vi "Sensor Simulation Initialization VI.vi"(8 "error in (no error)":errorcluster, 10 "Custom XML":string, 11 "Device Item Ref in":T1 format="%.0x") -> (0 "error out":errorcluster, 3 "Device Item Ref out":T1 format="%.0x")   [LabVIEW 2011, in "Sensor Simulation Custom Device.lvlib"]
uses:
  Sensor Simulation Custom Device.lvlib
  <vilib>/NI Veristand/Custom Device API/Custom Device Item Ref.ctl
  <vilib>/NI Veristand/Custom Device API/Dependent File Optional Info.ctl
  Real-Time/TypeDefs/SensorType.ctl
  <vilib>/NI Veristand/Custom Device API/Custom Device Channel.ctl
  <vilib>/NI Veristand/Custom Device API/Custom Device Channel Type.ctl
  Global.vi
  <vilib>/NI Veristand/Custom Device API/Set Item Property (Path).vi
  <vilib>/NI Veristand/Custom Device API/Set Item Property (String).vi
  <vilib>/NI Veristand/Custom Device API/Set Item Property (Boolean).vi
  <vilib>/NI Veristand/Custom Device API/Set Item Property (Dependent Node Pointer).vi
  <vilib>/NI Veristand/Custom Device API/Set Item Property (Dependent File).vi
  <vilib>/NI Veristand/Custom Device API/Set Item Property (Variant).vi
  <vilib>/NI Veristand/Custom Device API/Custom Device API.lvlib
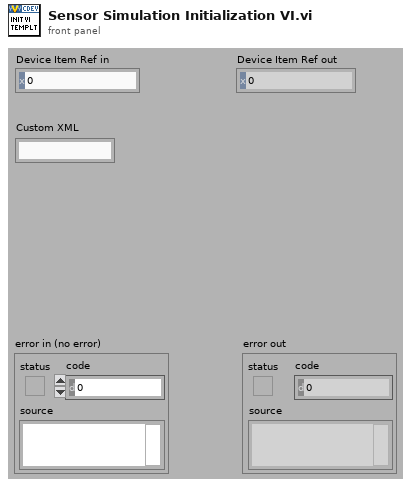
[diagram p1: front panel]
types:
  T1 = typedef "Custom Device API.lvlib/Custom Device Item Ref.ctl" = u64
  T2 = typedef "Sensor Simulation Custom Device.lvlib/SensorType.ctl" = enum16{"Resolver", "4 Wire xVDT", "5 Wire xVDT", "Invalid"}
  T3 = typedef "Custom Device API.lvlib/Custom Device Channel.ctl" = cluster{"Type":T4, "Units":string, "Default Value":dbl, "Faultable":bool, "Scalable":bool}
  T4 = typedef "Custom Device API.lvlib/Custom Device Channel Type.ctl" = enum16{"Input", "Output"}
  T5 = typedef "Custom Device API.lvlib/Dependent File Optional Info.ctl" = cluster{"Version":string, "RTDestination":path, "ForceDownload":bool, "SupportedTarget":string, "MD5":string}
  T6 = typedef "Sensor Simulation Custom Device.lvlib/SensorSimComps.ctl" = cluster{"xVDTs":T7[], "Resolvers":T8[]}
  T7 = typedef "Sensor Simulation Custom Device.lvlib/xVDT.ctl" = cluster{"ScaleFactor 1":string, "ScaleFactor 2":string, "#":string}
  T8 = typedef "Sensor Simulation Custom Device.lvlib/Resolver.ctl" = cluster{"ScaleFactor 1":string, "ScaleFactor 2":string, "#":string}
  T9 = cluster{"RIO Device Address":string, "Bitfile Signature":string, "Engine Sim Components":T6}
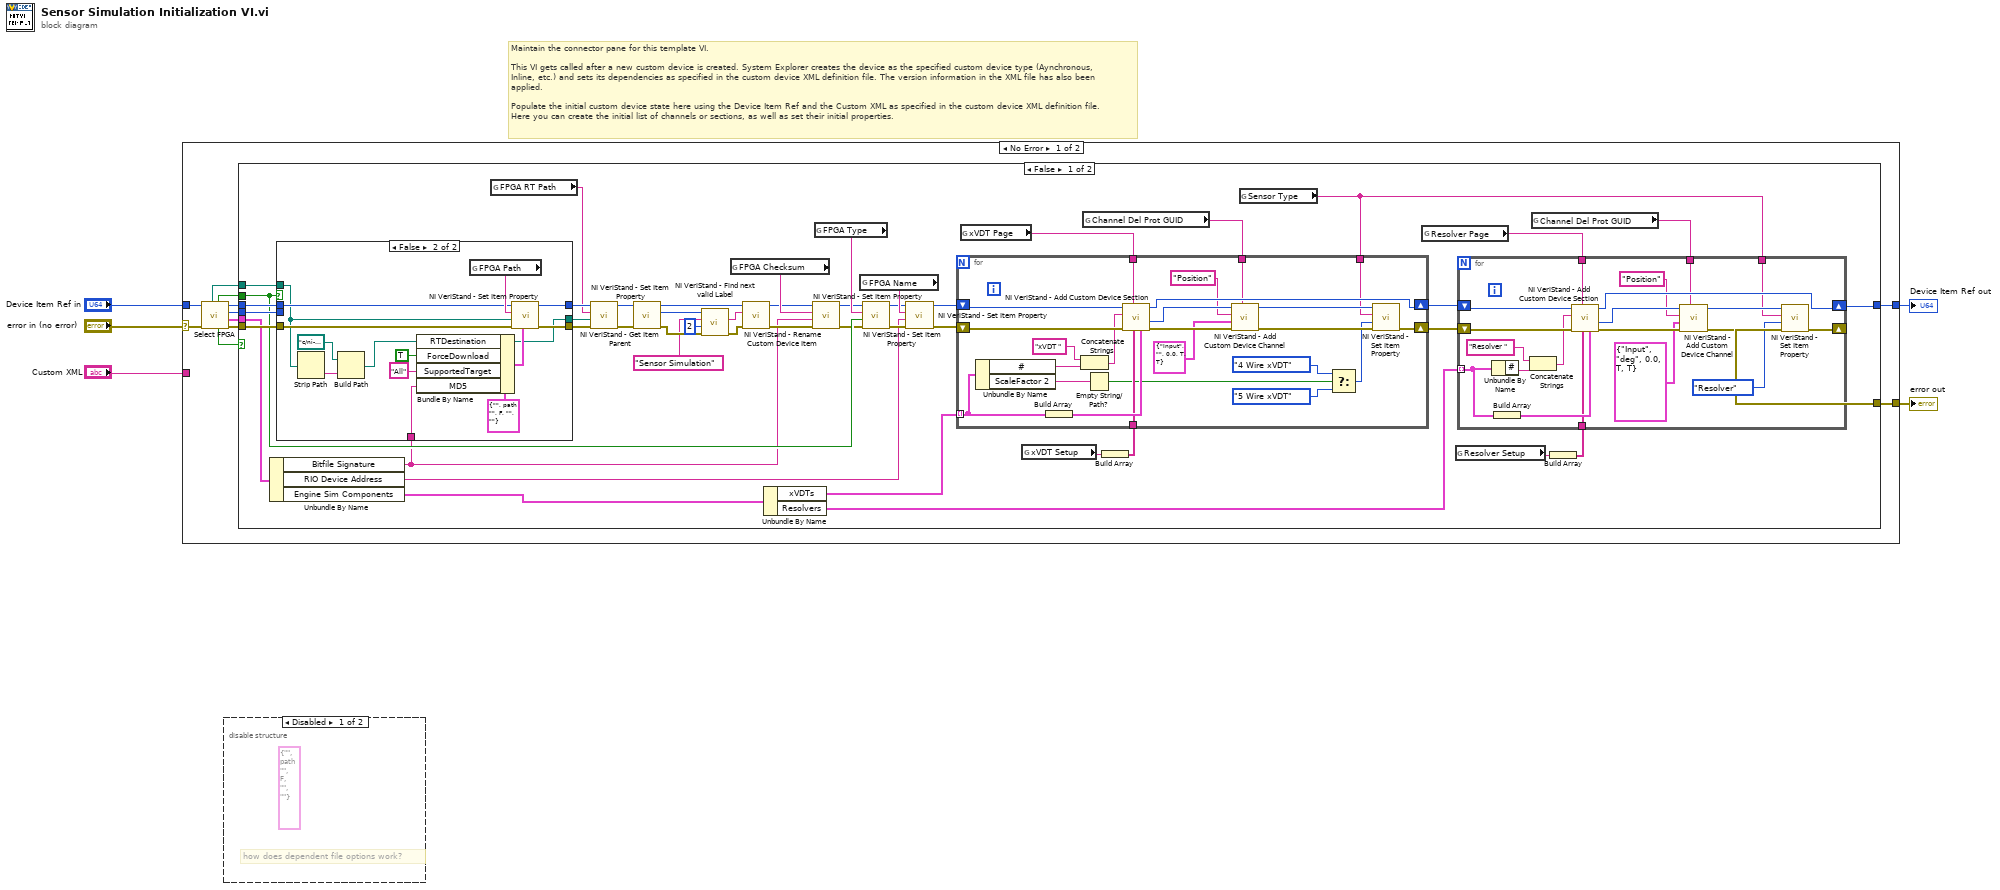
[diagram p0: block diagram]
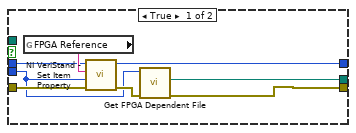
[diagram p3: hidden frame]
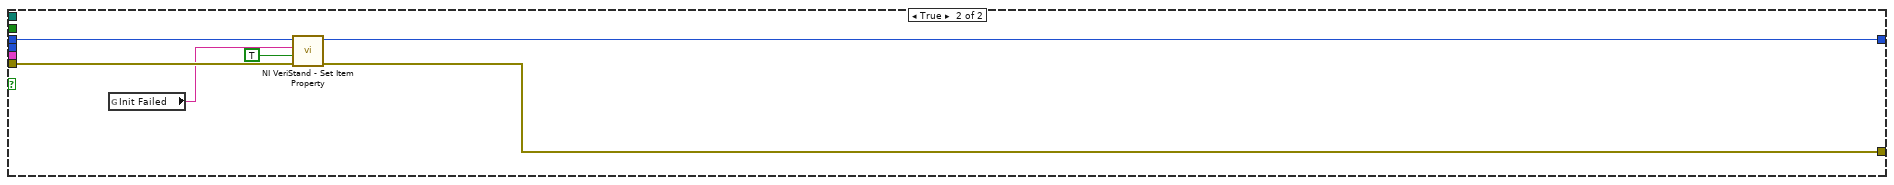
[diagram p4: hidden frame]
diagram:
  # "Maintain the connector pane for this template VI.\n\nThis VI gets called after a new custom device is created. System Explorer creates the device as the specified custom device type (Aynchronous, Inline, etc.) and sets its dependencies as specified in the custom device XML definition file. The version information in the XML file has also been applied.\n\nPopulate the initial custom device state here using the Device Item Ref and the Custom XML as specified in the custom device XML definition file. Here you can create the initial list of channels or sections, as well as set their initial properties."
  n1 = case shown="No Error" "error in (no error)" {
    selector: "error in (no error)" -> [w15 w136]
    tunnel: [w8 w136] -> w5
    tunnel: [w7 w135] -> w3
    tunnel: "Device Item Ref in" -> [w16 w135]
    tunnel: "Custom XML" -> [_ _]
    frame No Error {
      n2 = call "Select FPGA.vi"("error in"=w15, "Item Ref in"=w16) -> ("error out"=w13:errorcluster, "FPGA Info"=w11:T9, "FPGA Reference"=w14:T1, "Item Ref out"=w12:T1, "Cancelled?"=w6:bool, "VS FPGA?"=w10:bool, "Bitfile Path out"=w9:path)  [unwired: 3 in]
      n3 = case shown="False" w6 {
        tunnel: w14 -> [w62 _]
        tunnel: w13 -> [w61 w133]
        tunnel: w12 -> [w60 w134]
        tunnel: w11 -> [w59 _]
        tunnel: w10 -> [w58 _]
        tunnel: w9 -> [w57 _]
        tunnel: [w22 w132] -> w8
        tunnel: [w23 w131] -> w7
        frame False {
          n4 = Unbundle By Name(w59) -> ("Bitfile Signature"=w38:string, "RIO Device Address"=w48:string, "Engine Sim Components"=w56:T6)
          n5 = case shown="False" w58 {
            tunnel: w62 -> [w110 _]
            tunnel: w61 -> [w112 w126]
            tunnel: w60 -> [w113 w127]
            tunnel: w57 -> [_ w123]
            tunnel: [w109 w125] -> w20
            tunnel: [w108 w124] -> w19
            tunnel: w38 -> [_ w116]
            tunnel: [w107 w115] -> w18
            frame True {
              n6 = global read "Global.vi" "FPGA Reference"() -> (w114:string)
              n7 = call-poly <vilib>:"NI VeriStand - Set Item Property.vi"("error in (no error)"=w112, "Dependent Node Ref"=w110, "Property Name"=w114, "Item Ref in"=w113) -> ("error out"=w111:errorcluster, "Item Ref out"=w108:T1)  [unwired: 5 in, 1 out]
              n8 = call "Get FPGA Dependent File.vi"("error in (no error)"=w111, "ID in"=w110) -> ("error out"=w109:errorcluster, "RT Path"=w107:path)  [unwired: 7 in, 1 out]
            }
            frame False {
              n9 = Strip Path(path=w123) -> (name=w122:string)  [unwired: 1 out]
              n10 = Build Path(base path=path "c:/ni-rt/NIVeriStand/Custom Devices/Sensor Simulation" ("RTDestination"), name or relative path=w122) -> (appended path=w115:path)
              n11 = Bundle By Name(cluster=T5 {"Version"="", "RTDestination"=path "", "ForceDownload"=FALSE, "SupportedTarget"="", "MD5"=""} ("OptionalInfo"), "RTDestination"=w115, "ForceDownload"=TRUE, "SupportedTarget"="All", "MD5"=w116) -> (w118:T5)
              n12 = global read "Global.vi" "FPGA Path"() -> (w128:string)
              n13 = call-poly <vilib>:"NI VeriStand - Set Item Property.vi"("OptionalInfo"=w118, "error in (no error)"=w126, "Path"=w123, "Property Name"=w128, "Item Ref in"=w127) -> ("error out"=w125:errorcluster, "Item Ref out"=w124:T1)  [unwired: 4 in, 1 out]
            }
          }
          n14 = global read "Global.vi" "FPGA RT Path"() -> (w17:string)
          n15 = call-poly <vilib>:"NI VeriStand - Set Item Property.vi"("error in (no error)"=w20, "Value"=w18, "Property Name"=w17, "Item Ref in"=w19) -> ()  [unwired: 5 in, 3 out]
          n16 = call <vilib>:"NI VeriStand - Get Item Parent.vi"("error in (no error)"=w20, "Item Ref in"=w19) -> ("error out"=w42:errorcluster, "Parent Ref"=w44:T1, "Item Ref out"=w45:T1)  [unwired: 6 in, 1 out]
          n17 = call <vilib>:"NI VeriStand - Find next valid Label.vi"("error in (no error)"=w42, "Start Value (1)"=2, "Label"="Sensor Simulation", "Item Ref in"=w44) -> ("error out"=w41:errorcluster, "Label out"=w43:string)  [unwired: 3 in, 3 out]
          n18 = global read "Global.vi" "FPGA Checksum"() -> (w51:string)
          n19 = call <vilib>:"NI VeriStand - Rename Custom Device Item.vi"("error in (no error)"=w41, "New Name"=w43, "Item Ref in"=w45) -> ("error out"=w47:errorcluster, "Item Ref out"=w46:T1)  [unwired: 6 in, 1 out]
          n20 = Unbundle By Name(w56) -> ("xVDTs"=w37:T7[], "Resolvers"=w24:T8[])
          n21 = call-poly <vilib>:"NI VeriStand - Set Item Property.vi"("error in (no error)"=w47, "Value"=w38, "Property Name"=w51, "Item Ref in"=w46) -> ("error out"=w50:errorcluster, "Item Ref out"=w49:T1)  [unwired: 5 in, 1 out]
          n22 = global read "Global.vi" "FPGA Type"() -> (w52:string)
          n23 = global read "Global.vi" "FPGA Name"() -> (w55:string)
          n24 = call-poly <vilib>:"NI VeriStand - Set Item Property.vi"("error in (no error)"=w50, "Value"=w58, "Property Name"=w52, "Item Ref in"=w49) -> ("error out"=w53:errorcluster, "Item Ref out"=w54:T1)  [unwired: 5 in, 1 out]
          n25 = call-poly <vilib>:"NI VeriStand - Set Item Property.vi"("error in (no error)"=w53, "Value"=w48, "Property Name"=w55, "Item Ref in"=w54) -> ("error out"=w36:errorcluster, "Item Ref out"=w35:T1)  [unwired: 5 in, 1 out]
          n26 = global read "Global.vi" "xVDT Page"() -> (w34:string)
          n27 = global read "Global.vi" "xVDT Setup"() -> (w32:string)
          n28 = global read "Global.vi" "Channel Del Prot GUID"() -> (w33:string)
          n29 = Build Array(w32) -> (w31:string[])
          n30 = global read "Global.vi" "Sensor Type"() -> (w21:string)
          n31 = for {
            tunnel: w37 -> [w95] mode=indexing
            shift-right: [w86] -> w25
            shift-left: w36 -> [w106]
            tunnel: w34 -> [w104]
            tunnel: w33 -> [w96]
            tunnel: w31 -> [w93]
            shift-right: [w99] -> w26
            shift-left: w35 -> [w105]
            tunnel: w21 -> [w87]
            n32 = Unbundle By Name(w95) -> ("#"=w92:string, "ScaleFactor 2"=w91:string)
            n33 = Build Array(w95) -> (w94:T7[])
            n34 = Concatenate Strings("xVDT " ("string"), w92) -> (w102:string)
            n35 = Empty String/Path?(string/path=w91) -> (empty?=w90:bool)
            n36 = call <vilib>:"NI VeriStand - Add Custom Device Section.vi"("Property Values"=w94, "Property names"=w93, "GUID (Default Section)"=w104, "error in (no error)"=w106, "Section Name"=w102, "Parent Ref in"=w105) -> ("error out"=w101:errorcluster, "Section Ptr"=w100:T1, "Parent Ref out"=w99:T1)  [unwired: 2 in, 1 out]
            n37 = call <vilib>:"NI VeriStand - Add Custom Device Channel.vi"("GUID (Default Channel)"=w96, "error in (no error)"=w101, "Channel"=T3 {"Type"=enum."Input", "Units"="", "Default Value"=0.0, "Faultable"=TRUE, "Scalable"=TRUE}, "Channel Name"="Position", "Parent Ref in"=w100) -> ("error out"=w88:errorcluster, "Parent Ref out"=w89:T1)  [unwired: 3 in, 2 out]
            n38 = Select(t=SensorType."4 Wire xVDT" ("Sensor"), s=w90, f=SensorType."5 Wire xVDT" ("Sensor")) -> (s? t:f=w83:T2)
            n39 = call-poly <vilib>:"NI VeriStand - Set Item Property.vi"("error in (no error)"=w88, "Value"=w83, "Property Name"=w87, "Item Ref in"=w89) -> ("error out"=w86:errorcluster)  [unwired: 5 in, 2 out]
          }
          n40 = global read "Global.vi" "Resolver Page"() -> (w27:string)
          n41 = global read "Global.vi" "Resolver Setup"() -> (w29:string)
          n42 = global read "Global.vi" "Channel Del Prot GUID"() -> (w28:string)
          n43 = Build Array(w29) -> (w30:string[])
          n44 = for {
            tunnel: w24 -> [w72] mode=indexing
            shift-right: [w64] -> w22
            shift-left: w25 -> [w82]
            tunnel: w27 -> [w80]
            tunnel: w28 -> [w73]
            tunnel: w30 -> [w70]
            shift-right: [w76] -> w23
            shift-left: w26 -> [w81]
            tunnel: w21 -> [w65]
            n45 = Unbundle By Name(w72) -> ("#"=w69:string)
            n46 = Build Array(w72) -> (w71:T8[])
            n47 = Concatenate Strings("Resolver " ("string"), w69) -> (w79:string)
            n48 = call <vilib>:"NI VeriStand - Add Custom Device Section.vi"("Property Values"=w71, "Property names"=w70, "GUID (Default Section)"=w80, "error in (no error)"=w82, "Section Name"=w79, "Parent Ref in"=w81) -> ("error out"=w78:errorcluster, "Section Ptr"=w77:T1, "Parent Ref out"=w76:T1)  [unwired: 2 in, 1 out]
            n49 = call <vilib>:"NI VeriStand - Add Custom Device Channel.vi"("GUID (Default Channel)"=w73, "error in (no error)"=w78, "Channel"=T3 {"Type"=enum."Input", "Units"="deg", "Default Value"=0.0, "Faultable"=TRUE, "Scalable"=TRUE}, "Channel Name"="Position", "Parent Ref in"=w77) -> ("error out"=w67:errorcluster, "Parent Ref out"=w66:T1)  [unwired: 3 in, 2 out]
            n50 = call-poly <vilib>:"NI VeriStand - Set Item Property.vi"("error in (no error)"=w67, "Value"=SensorType."Resolver" ("Sensor"), "Property Name"=w65, "Item Ref in"=w66) -> ("error out"=w64:errorcluster)  [unwired: 5 in, 2 out]
          }
        }
        frame True {
          n51 = global read "Global.vi" "Init Failed"() -> (w129:string)
          n52 = call-poly <vilib>:"NI VeriStand - Set Item Property.vi"("error in (no error)"=w133, "Value"=TRUE, "Property Name"=w129, "Item Ref in"=w134) -> ("error out"=w132:errorcluster, "Item Ref out"=w131:T1)  [unwired: 5 in, 1 out]
        }
      }
    }
    frame Error {
    }
  }
  "error out" <- w5
  "Device Item Ref out" <- w3
  n53 = disable-structure shown="Disabled" {
    frame Disabled {
      (unwired) T5 {"Version"="", "RTDestination"=path "", "ForceDownload"=FALSE, "SupportedTarget"="", "MD5"=""} ("OptionalInfo")
      # "how does dependent file options work?"
    }
    frame Enabled {
    }
  }
